vi "Robot State (Global Variable).vi"() -> ()   [LabVIEW 2018]
uses:
  Controls/Robot State.ctl
  Controls/Robot Pivot Motion Commands.ctl
  Controls/Pivot Motor Commands.ctl
  Controls/Robot Drive Mode.ctl
  Controls/Climb Motor Commands.ctl
  Controls/Arm Motor Commands.ctl
  Controls/Ball Motor Commands.ctl
  Controls/Dics Eject Command.ctl
  Controls/Lift Motor Commands.ctl
  Controls/Grip Motor Commands.ctl
  Controls/Enable Actions.ctl
panel:
  out "Robot State":T1
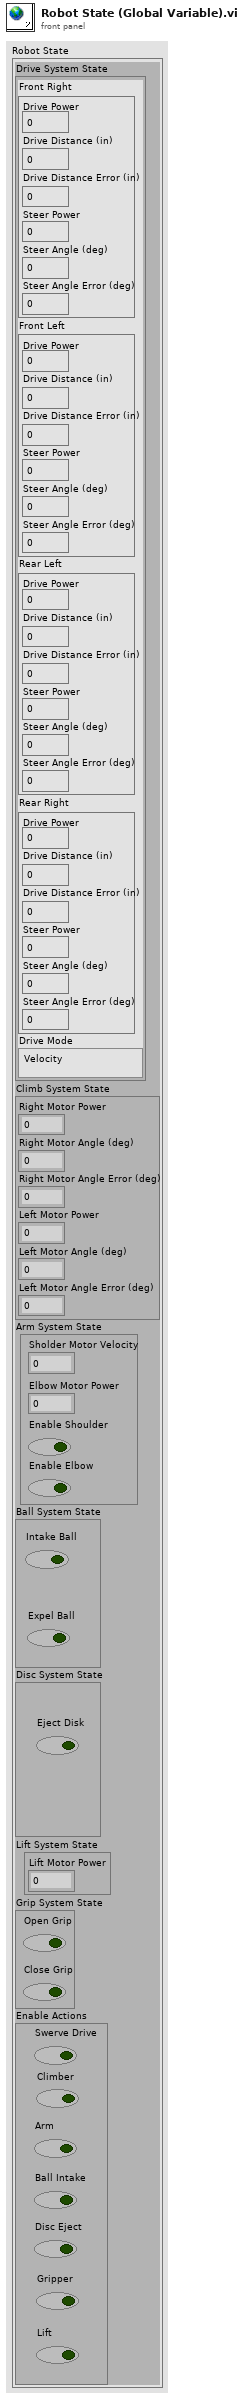
[diagram p1: front panel]
types:
  T1 = typedef "Robot State.ctl" = cluster{"Drive System State":T2, "Climb System State":T5, "Arm System State":T6, "Ball System State":T7, "Disc System State":T8, "Lift System State":T9, "Grip System State":T10, "Enable Actions":T11}
  T2 = typedef "Robot Pivot Motion Commands.ctl" = cluster{"Front Right":T3, "Front Left":T3, "Rear Left":T3, "Rear Right":T3, "Drive Mode":T4}
  T3 = typedef "Pivot Motor Commands.ctl" = cluster{"Drive Power":dbl, "Drive Distance (in)":dbl, "Drive Distance Error (in)":dbl, "Steer Power":dbl, "Steer Angle (deg)":dbl, "Steer Angle Error (deg)":dbl}
  T4 = typedef "Robot Drive Mode.ctl" = enum16{"Velocity", "Distance"}
  T5 = typedef "Climb Motor Commands.ctl" = cluster{"Right Motor Power":dbl, "Right Motor Angle (deg)":dbl, "Right Motor Angle Error (deg)":dbl, "Left Motor Power":dbl, "Left Motor Angle (deg)":dbl, "Left Motor Angle Error (deg)":dbl}
  T6 = typedef "Arm Motor Commands.ctl" = cluster{"Enable Shoulder":bool, "Enable Elbow":bool, "Elbow Motor Power":dbl, "Sholder Motor Velocity":dbl}
  T7 = typedef "Ball Motor Commands.ctl" = cluster{"Intake Ball":bool, "Expel Ball":bool}
  T8 = typedef "Dics Eject Command.ctl" = cluster{"Eject Disk":bool}
  T9 = typedef "Lift Motor Commands.ctl" = cluster{"Lift Motor Power":dbl}
  T10 = typedef "Grip Motor Commands.ctl" = cluster{"Open Grip":bool, "Close Grip":bool}
  T11 = typedef "Enable Actions.ctl" = cluster{"Swerve Drive":bool, "Climber":bool, "Arm":bool, "Ball Intake":bool, "Disc Eject":bool, "Gripper":bool, "Lift":bool}
diagram:
